vi "CCD ReadoutBytes.vi"(0 "CCD Setup String":string="ldB,1,53,u,0,150,25,B,1,53;sdu,0,1024,1024;cl2;omrm;sron") -> (2 "RM(T) or RT(F) mode":bool, 3 "Bytes for Readout":i32=51201, 4 "LD Bytes":i32=25, 5 "SD Bytes":i32=1024)   [LabVIEW 2020]
doc: "converrts the CCD setup string into the amount of bytes \nto be read. Eaxmple:\n ldu,0,256,16;sdu0,1024,1024;...;...;...\nyields: ((16[LD]*1024[SD])*2)+1 bytes"
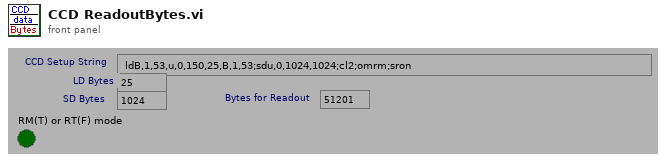
[diagram p1: front panel]
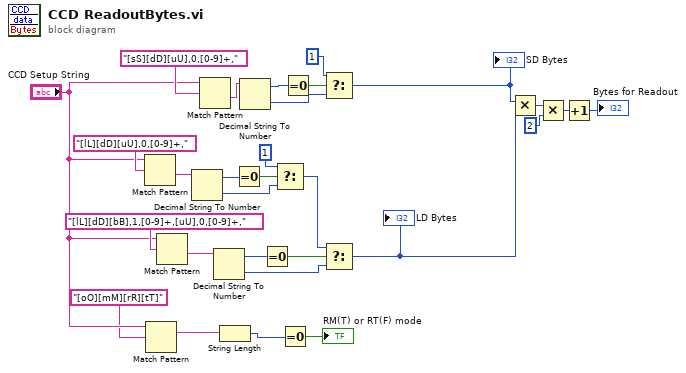
[diagram p0: block diagram]
diagram:
  n1 = Match Pattern(string="CCD Setup String", regular expression="[lL][dD][uU],0,[0-9]+,") -> (after substring=w11:string)  [unwired: 1 in, 3 out]
  n2 = Match Pattern(string="CCD Setup String", regular expression="[oO][mM][rR][tT]") -> (match substring=w3:string)  [unwired: 1 in, 3 out]
  n3 = Match Pattern(string="CCD Setup String", regular expression="[lL][dD][bB],1,[0-9]+,[uU],0,[0-9]+,") -> (after substring=w19:string)  [unwired: 1 in, 3 out]
  n4 = Decimal String To Number(string=w11) -> (offset past number=w9:i32, number=w8:i32)  [unwired: 2 in]
  n5 = Match Pattern(string="CCD Setup String", regular expression="[sS][dD][uU],0,[0-9]+,") -> (after substring=w20:string)  [unwired: 1 in, 3 out]
  n6 = Decimal String To Number(string=w19) -> (offset past number=w21:i32, number=w22:i32)  [unwired: 2 in]
  n7 = String Length(string=w3) -> (length=w2:i32)
  n8 = Equal To 0?(x=w9) -> (x = 0?=w10:bool)
  n9 = Decimal String To Number(string=w20) -> (offset past number=w27:i32, number=w24:i32)  [unwired: 2 in]
  n10 = Equal To 0?(x=w21) -> (x = 0?=w25:bool)
  n11 = Select(t=1, s=w10, f=w8) -> (s? t:f=w6:i32)
  n12 = Equal To 0?(x=w2) -> (x = 0?=→"RM(T) or RT(F) mode":bool)
  n13 = Equal To 0?(x=w27) -> (x = 0?=w26:bool)
  n14 = Select(t=1, s=w26, f=w24) -> (s? t:f=w17:i32)
  "SD Bytes" <- w17
  n15 = Select(t=w6, s=w25, f=w22) -> (s? t:f=w16:i32)
  "LD Bytes" <- w16
  n16 = Multiply(x=w17, y=w16) -> (x*y=w14:i32)
  n17 = Multiply(x=w14, y=2) -> (x*y=w15:i32)
  n18 = Increment(x=w15) -> (x+1=→"Bytes for Readout":i32)
